vi "Periodic Tasks.vi"(8 "error in":errorcluster) -> ()   [LabVIEW 2019]
doc: "This VI runs in parallel to other tasks. It can contain as many user-defined periodic loops as you need. These can carry out PID or other sorts of timed response."
panel:
  in  "Milliseconds between threshold":dbl
  in  "threshold":dbl=0.05
  out "IsDisconnected?":bool
  in  "VoltageWhenUnplugged":dbl=0.24
  out "Voltage":dbl
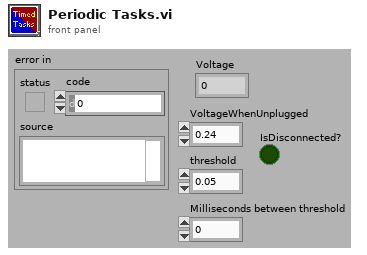
[diagram p1: front panel]
types:
  T1 = typedef "WPI_AnalogChannelDevRef.ctl" = cluster{"DevStatus":errorcluster, "Analog Channel":T2}
  T2 = typedef "FPGA_AIChannel.ctl" = enum8{"AI 0", "AI 1", "AI 2", "AI 3", "AI MXP 0", "AI MXP 1", "AI MXP 2", "AI MXP 3", "Invalid"}
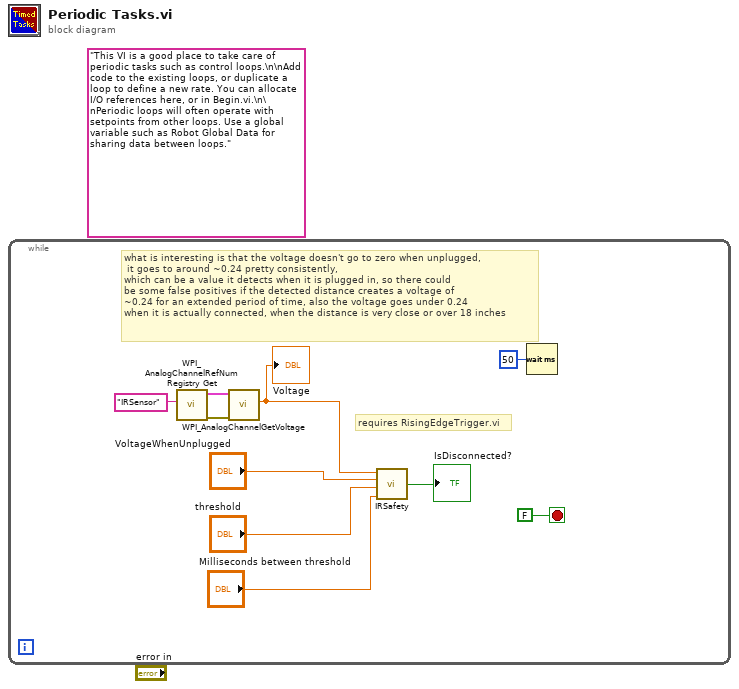
[diagram p0: block diagram]
diagram:
  (unwired) "This VI is a good place to take care of periodic tasks such as control loops.\n\nAdd code to the existing loops, or duplicate a loop to define a new rate. You can allocate I/O references here, or in Begin.vi.\n\nPeriodic loops will often operate with setpoints from other loops. Use a global variable such as Robot Global Data for sharing data between loops."
  n1 = while {
    stop <- FALSE stop-if-true
    # "requires RisingEdgeTrigger.vi"
    # "what is interesting is that the voltage doesn't go to zero when unplugged,\n it goes to around ~0.24 pretty consistently,\nwhich can be a value it detects when it is plugged in, so there could \nbe some false positives if the detected distance creates a voltage of \n~0.24 for an extended period of time, also the voltage goes under 0.24\nwhen it is actually connected, when the distance is very close or over 18 inches"
    n2 = call <vilib>:"WPI_AnalogChannelRefNum Registry Get.vi"("refnum name"="IRSensor") -> ("error out"=w7:errorcluster, "AIDeviceRef"=w8:T1)  [unwired: 9 in]
    n3 = call <vilib>:"WPI_AnalogChannelGetVoltage.vi"("error in (no error)"=w7, "AIDeviceRef"=w8) -> ("Voltage"=w4:dbl)  [unwired: 7 in, 2 out]
    "Voltage" <- w4
    n4 = call "IRSafety.vi"("MillisecondsBetweenThreshold"="Milliseconds between threshold", "threshold"="threshold", "VoltageWhenUnplugged"="VoltageWhenUnplugged", "Voltage"=w4) -> ("Boolean"=→"IsDisconnected?":bool)
    n5 = Wait (ms)(milliseconds to wait=u32 50) -> ()  [unwired: 1 out]
  }
